vi "sftp_error.vi"() -> ()   [LabVIEW 2013]
doc: "Illustrates how to handle errors when using SFTP."
uses:
  <vilib>/Utility/error.llb/DialogType.ctl
  libssh2/libssh2_init_default.vi
  libssh2/libssh2_session_handshake_tcp.vi
  libssh2/libssh2.lvlib
panel:
  out "error out":errorcluster
  in  "password":string
  in  "username":string
  in  "hostname":string
  # "This example, when executed, will return a missing-file error."
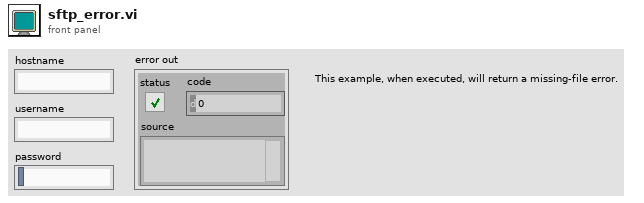
[diagram p1: front panel]
types:
  T1 = typedef "DialogType.ctl" = u16
  T2 = typedef "libssh2.lvlib/Session Refnum.ctl" = refnum<k1>
  T3 = typedef "libssh2.lvlib/SFTP Refnum.ctl" = refnum<k1>
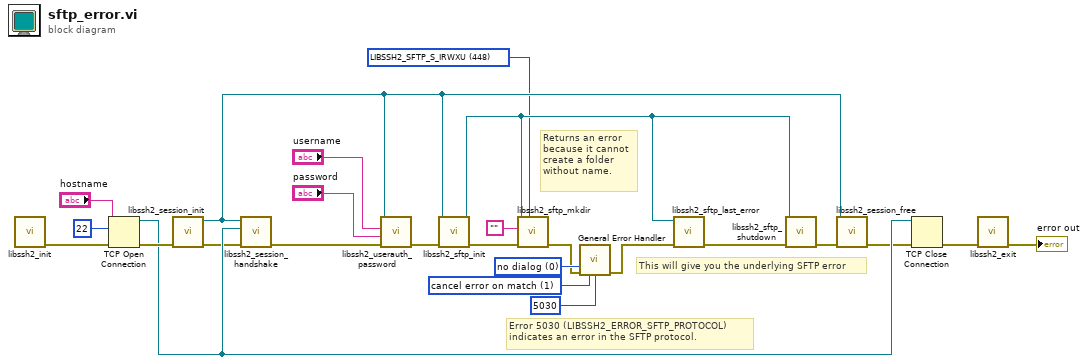
[diagram p0: block diagram]
diagram:
  w4 = T1 0 items=["no dialog", "OK message", "continue or stop message", "OK message + warnings", "continue/stop + warnings"] ("type of dialog (OK msg:1)")
  w6 = 1 items=["no exception", "cancel error on match", "set error on match"] ("[exception action] (none:0)")
  w7 = 448 items=["LIBSSH2_SFTP_S_IRWXU"=448, "LIBSSH2_SFTP_S_IRUSR"=256, "LIBSSH2_SFTP_S_IWUSR"=128, "LIBSSH2_SFTP_S_IXUSR"=64, "LIBSSH2_SFTP_S_IRWXG"=56, "LIBSSH2_SFTP_S_IRGRP"=32, "LIBSSH2_SFTP_S_IWGRP"=16, "LIBSSH2_SFTP_S_IXGRP"=8, "LIBSSH2_SFTP_S_IRWXO"=7, "LIBSSH2_SFTP_S_IROTH"=4, "LIBSSH2_SFTP_S_IWOTH"=2, "LIBSSH2_SFTP_S_IXOTH"=1] ("mode")
  # "This will give you the underlying SFTP error"
  # "Error 5030 (LIBSSH2_ERROR_SFTP_PROTOCOL)\nindicates an error in the SFTP protocol."
  # "Returns an error\nbecause it cannot\ncreate a folder\nwithout name."
  n1 = call-poly "libssh2_init.vi"() -> ("error out"=w24:errorcluster)  [unwired: 11 in]
  n2 = TCP Open Connection(address="hostname", remote port or service name=u16 22, error in (no error)=w24) -> (connection ID=w22:refnum<k5>, error out=w23:errorcluster)  [unwired: 2 in]
  n3 = call "libssh2_session_init.vi"("error in (no error)"=w23) -> ("error out"=w21:errorcluster, "session"=w14:T2)  [unwired: 9 in]
  n4 = call-poly "libssh2_session_handshake.vi"("error in (no error)"=w21, "tcp connection"=w22, "session"=w14) -> ("error out"=w25:errorcluster)  [unwired: 8 in]
  n5 = call "libssh2_userauth_password.vi"("error in (no error)"=w25, "password"="password", "username"="username", "session"=w14) -> ("error out"=w18:errorcluster)  [unwired: 7 in]
  n6 = call "libssh2_sftp_init.vi"("error in (no error)"=w18, "session"=w14) -> ("error out"=w10:errorcluster, "sftp"=w9:T3)  [unwired: 8 in]
  n7 = call "libssh2_sftp_mkdir.vi"("mode"=w7, "error in (no error)"=w10, "path"="" ("file"), "sftp"=w9) -> ("error out"=w3:errorcluster)  [unwired: 7 in]
  n8 = call <vilib>:"General Error Handler.vi"("type of dialog (OK msg:1)"=w4, "error in (no error)"=w3, "[exception action] (none:0)"=w6, "[exception code]"=5030 ("specific error code to clear (0: all)")) -> ("error out"=w2:errorcluster)  [unwired: 7 in, 4 out]
  n9 = call "libssh2_sftp_last_error.vi"("error in (no error)"=w2, "sftp"=w9) -> ("error out"=w1:errorcluster)  [unwired: 9 in]
  n10 = call "libssh2_sftp_shutdown.vi"("error in (no error)"=w1, "sftp"=w9) -> ("error out"=w11:errorcluster)  [unwired: 9 in]
  n11 = call "libssh2_session_free.vi"("error in (no error)"=w11, "session"=w14) -> ("error out"=w13:errorcluster)  [unwired: 9 in]
  n12 = TCP Close Connection(connection ID=w22, error in (no error)=w13) -> (error out=w12:errorcluster)  [unwired: 1 in, 1 out]
  n13 = call "libssh2_exit.vi"("error in (no error)"=w12) -> ("error out"=→"error out":errorcluster)  [unwired: 10 in]
